vi "ConfigureMDrive.vi"(0 "Address":u8, 1 "Port Name":string, 2 "ConfigString":string, 3 "Channel Name":string) -> (8 "Good Echo":bool)   [LabVIEW 2010]
panel:
  out "Array 2":string[](array[string])
  out "Array":bool[](array[boolean])
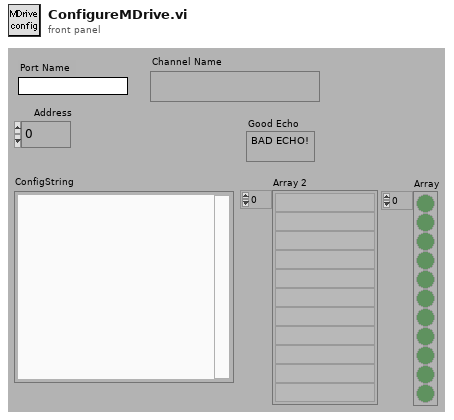
[diagram p1: front panel]
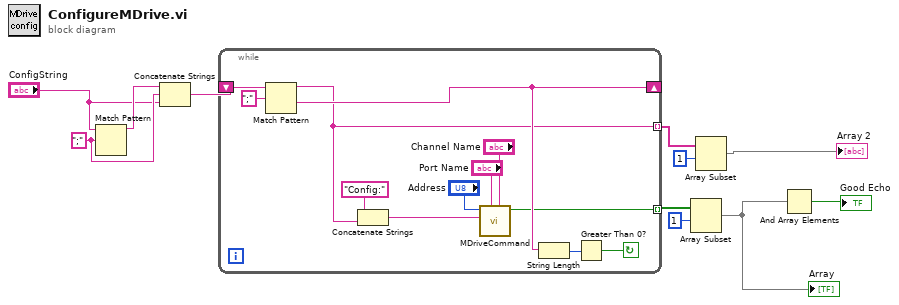
[diagram p0: block diagram]
diagram:
  w9 = ";" ("regular expression")
  n1 = Match Pattern(string="ConfigString", regular expression=w9) -> (before substring=w10:string)  [unwired: 4 out]
  n2 = Concatenate Strings(w10, w9, "ConfigString") -> (w11:string)
  n3 = while {
    shift-right: [w14] -> _
    shift-left: w11 -> [w20]
    tunnel: [w13] -> w8 mode=indexing
    tunnel: [w12] -> w4 mode=indexing
    stop <- w16 continue-if-true
    n4 = Match Pattern(string=w20, regular expression=";") -> (before substring=w12:string, after substring=w14:string)  [unwired: 3 out]
    n5 = Concatenate Strings("Config:" ("string"), w12) -> (w17:string)
    n6 = call "MDriveCommand.vi"("Channel Name"="Channel Name", "Port Name"="Port Name", "MDriveCommand"=w17, "Address"="Address") -> ("OK"=w13:bool)  [unwired: 1 in, 5 out]
    n7 = String Length(string=w14) -> (length=w15:i32)
    n8 = Greater Than 0?(x=w15) -> (x > 0?=w16:bool)
  }
  n9 = Array Subset(array=w8, index=1) -> (w6:bool[])  [unwired: 1 in]
  "Array" <- w6
  n10 = Array Subset(array=w4, index=1) -> (→"Array 2":string[])  [unwired: 1 in]
  n11 = And Array Elements(Boolean array=w6) -> (logical AND=→"Good Echo":bool)
